vi "Hole_Center.vi"(8 "error in (no error)":errorcluster, 10 "Image In":T2, 11 "ROI Descriptor":T1 {"Contours"."Type" items=["No Selection", "Point", "Line", "Rectangle", "Oval", "Polygon", "Freehand Region", "Annulus", "Unused2", "Unused3", "Broken Line", "Freehand Line", "Rotated Rectangle"]}) -> (0 "error out":errorcluster, 1 "Center X &Y":cluster{"Center X":dbl, "Center Y":dbl}, 3 "Image Out":T2(plugin-control))   [LabVIEW 2019, in "Algorithm.lvclass"]
uses:
  FrameworkOverrides/Algorithm.lvclass
  <vilib>/vision/NI_Vision_Development_Module.lvlib
  <vilib>/vision/Image Controls.llb/IMAQ Image.ctl
panel:
  out "Binary Image":T2(plugin-control)
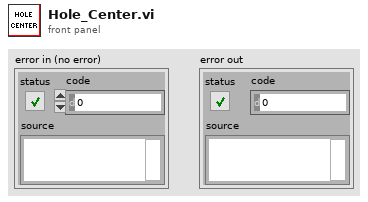
[diagram p1: front panel]
types:
  T1 = typedef "ROI Descriptor" = cluster{"Global Rectangle":i32[], "Contours":cluster{"ID":enum32{"External", "Internal"}, "Type":u32, "Coordinates":i32[]}[]}
  T2 = typedef "IMAQ Image.ctl" = refnum<image>
  T3 = typedef "Particle Parameters" = i32
  T4 = cluster{"Measurement Parameter":T3, "Range Lower Value":dbl, "Range Upper Value":dbl, "Range":bool, "Measurement Type":bool}[]
  T5 = typedef "Image Type" = u32
  T6 = typedef "IMAQ Rectangle" = cluster{"Left":i32, "Top":i32, "Right":i32, "Bottom":i32, "Rotation":dbl}
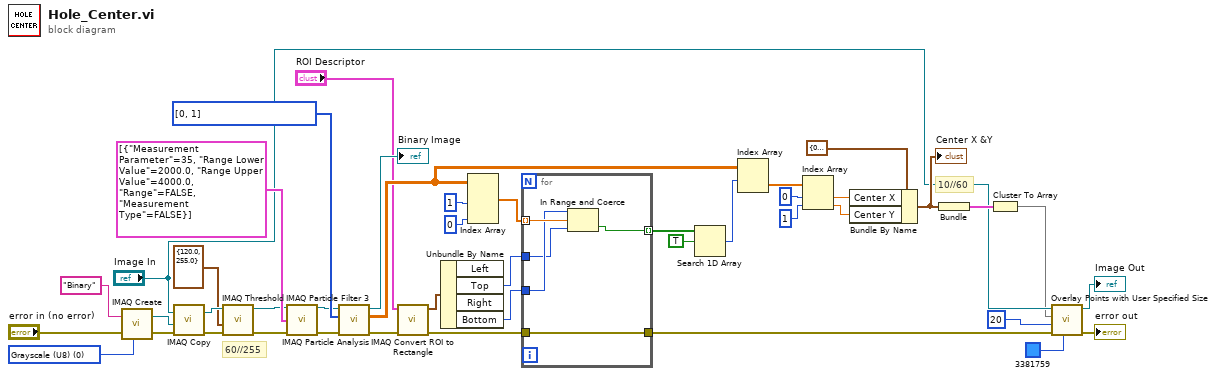
[diagram p0: block diagram]
diagram:
  w41 = T3[] [0, 1] items=["Center of Mass X", "Center of Mass Y", "First Pixel X", "First Pixel Y", "Bounding Rect Left", "Bounding Rect Top", "Bounding Rect Right", "Bounding Rect Bottom", "Max Feret Diameter Start X", "Max Feret Diameter Start Y", "Max Feret Diameter End X", "Max Feret Diameter End Y", "Max Horiz. Segment Length Left", "Max Horiz. Segment Length Right", "Max Horiz. Segment Length Row", "-", "Bounding Rect Width", "Bounding Rect Height", "Bounding Rect Diagonal", "Perimeter", "Convex Hull Perimeter", "Holes' Perimeter", "Max Feret Diameter", "Equivalent Ellipse Major Axis", "Equivalent Ellipse Minor Axis", "Equivalent Ellipse Minor Axis (Feret)", "Equivalent Rect Long Side", "Equivalent Rect Short Side", "Equivalent Rect Diagonal", "Equivalent Rect Short Side (Feret)", "Average Horiz. Segment Length", "Average Vert. Segment Length", "Hydraulic Radius", "Waddel Disk Diameter", "-", "Area", "Holes' Area", "Particle & Holes' Area", "Convex Hull Area", "Image Area", "-", "Number of Holes", "Number of Horiz. Segments", "Number of Vert. Segments", "-", "Orientation", "Max Feret Diameter Orientation", "-", "% Area/Image Area", "% Area/(Particle & Holes' Area)", "Ratio of Equivalent Ellipse Axes", "Ratio of Equivalent Rect Sides", "-", "Elongation Factor", "Compactness Factor", "Heywood Circularity Factor", "Type Factor", "-", "Sum X", "Sum Y", "Sum XX", "Sum XY", "Sum YY", "Sum XXX", "Sum XXY", "Sum XYY", "Sum YYY", "-", "Moment of Inertia XX", "Moment of Inertia XY", "Moment of Inertia YY", "Moment of Inertia XXX", "Moment of Inertia XXY", "Moment of Inertia XYY", "Moment of Inertia YYY", "Norm. Moment of Inertia XX", "Norm. Moment of Inertia XY", "Norm. Moment of Inertia YY", "Norm. Moment of Inertia XXX", "Norm. Moment of Inertia XXY", "Norm. Moment of Inertia XYY", "Norm. Moment of Inertia YYY", "Hu Moment 1", "Hu Moment 2", "Hu Moment 3", "Hu Moment 4", "Hu Moment 5", "Hu Moment 6", "Hu Moment 7"] ("Pixel Measurements")
  w36 = T5 0 items=["Grayscale (U8)", "Grayscale (I16)", "Grayscale (SGL)", "Complex (CSG)", "RGB (U32)", "HSL (U32)", "RGB (U64)", "Grayscale (U16)"] ("Image Type")
  # "10//60"
  # "60//255"
  n1 = call "IMAQ Create"("Image Name"="Binary", "Image Type"=w36, "error in (no error)"="error in (no error)") -> ("New Image"=w37:T2, "error out"=w5:errorcluster)  [unwired: 2 in]
  n2 = call "IMAQ Copy"("error in (no error)"=w5, "Image Dst"=w37, "Image Src"="Image In") -> ("error out"=w42:errorcluster, "Image Dst Out"=w43:T2)  [unwired: 3 in]
  n3 = call "IMAQ Threshold"("error in (no error)"=w42, "Range"=cluster{"Lower value":sgl, "Upper value":sgl} {"Lower value"=120.0, "Upper value"=255.0}, "Image Src"=w43) -> ("error out"=w21:errorcluster, "Image Dst Out"=w20:T2)  [unwired: 7 in]
  n4 = call "IMAQ Particle Filter 3"("Image Src"=w20, "Selection Values"=T4 [{"Measurement Parameter"=35, "Range Lower Value"=2000.0, "Range Upper Value"=4000.0, "Range"=FALSE, "Measurement Type"=FALSE}], "error in (no error)"=w21) -> ("Image Dst Out"=w39:T2, "error out"=w40:errorcluster)  [unwired: 10 in, 1 out]
  n5 = call "IMAQ Particle Analysis"("error in (no error)"=w40, "Pixel Measurements"=w41, "Image"=w39) -> ("error out"=w3:errorcluster, "Particle Measurements (Pixels)"=w25:dbl[][], "Image Out (duplicate)"=→"Binary Image":T2)  [unwired: 3 in, 3 out]
  n6 = call "IMAQ Convert ROI to Rectangle"("error in (no error)"=w3, "ROI Descriptor"="ROI Descriptor") -> ("error out"=w15:errorcluster, "Rectangle"=w18:T6)  [unwired: 7 in]
  n7 = Unbundle By Name(w18) -> ("Top"=w17:i32, "Bottom"=w16:i32)  [unwired: 2 out]
  n8 = Index Array(array=w25, index (col) #1=1 ("disabled index (col)"), index (col) #2=0 ("index (col)")) -> (element #1=w32:dbl[])  [unwired: 2 in, 1 out]
  n9 = for {
    tunnel: w32 -> [w48] mode=indexing
    tunnel: [w44] -> w31 mode=indexing
    tunnel: w16 -> [w47]
    tunnel: w17 -> [w46]
    tunnel: w15 -> [w45]
    tunnel: [w45] -> w14
    n10 = In Range and Coerce(upper limit=w47, x=w48, lower limit=w46) -> (In Range?=w44:bool)  [unwired: 1 out]
  }
  n11 = Search 1D Array(1D array=w31, element=TRUE) -> (index of element=w29:i32)  [unwired: 1 in]
  n12 = Index Array(array=w25, index (row)=w29) -> (element=w28:dbl[])  [unwired: 1 in]
  n13 = Index Array(array=w28, index #1=0 ("index"), index #2=1 ("index")) -> (element #1=w24:dbl, element #2=w23:dbl)
  n14 = Bundle By Name(cluster=cluster{"Center X":dbl, "Center Y":dbl} {"Center X"=0.0, "Center Y"=0.0}, "Center X"=w24, "Center Y"=w23) -> (w9:cluster{"Center X":dbl, "Center Y":dbl})
  "Center X &Y" <- w9
  n15 = Bundle(w9) -> (w12:cluster{cluster{"Center X":dbl, "Center Y":dbl}})  [unwired: 1 in]
  n16 = Cluster To Array(cluster=w12) -> (array=w1:cluster{"Center X":dbl, "Center Y":dbl}[])
  n17 = call "Overlay Points with User Specified Size.vi"("Color"=u32 3381759, "error in"=w14, "Point Diameter (5)"=u32 20, "Points"=w1, "Image In"="Image In") -> ("error out"=→"error out":errorcluster, "Image Out"=→"Image Out":T2)  [unwired: 5 in]
